vi "Get Feature Names.vi"(8 "error in (no error)":errorcluster caption="entrée d'erreur (pas d'erreur)", 9 "y":string[][](array[string]), 10 "X":string[][](array[string]), 11 "OneHotEncoder.lvclass":refnum<class "OneHotEncoder.lvclass">) -> (0 "error out":errorcluster caption="sortie d'erreur", 2 "Data":T1, 3 "OneHotEncoder.lvclass":refnum<class "OneHotEncoder.lvclass">)   [LabVIEW 2020, in "OneHotEncoder.lvclass"]
doc: "Return feature names for output features.\n\nReturns : \n\n- output_feature_names : ndarray of shape (n_output_features,)\nArray of feature names."
uses:
  OneHotEncoder.lvclass
  OneHotEncoder.lvclass/OneHotEncoder.ctl
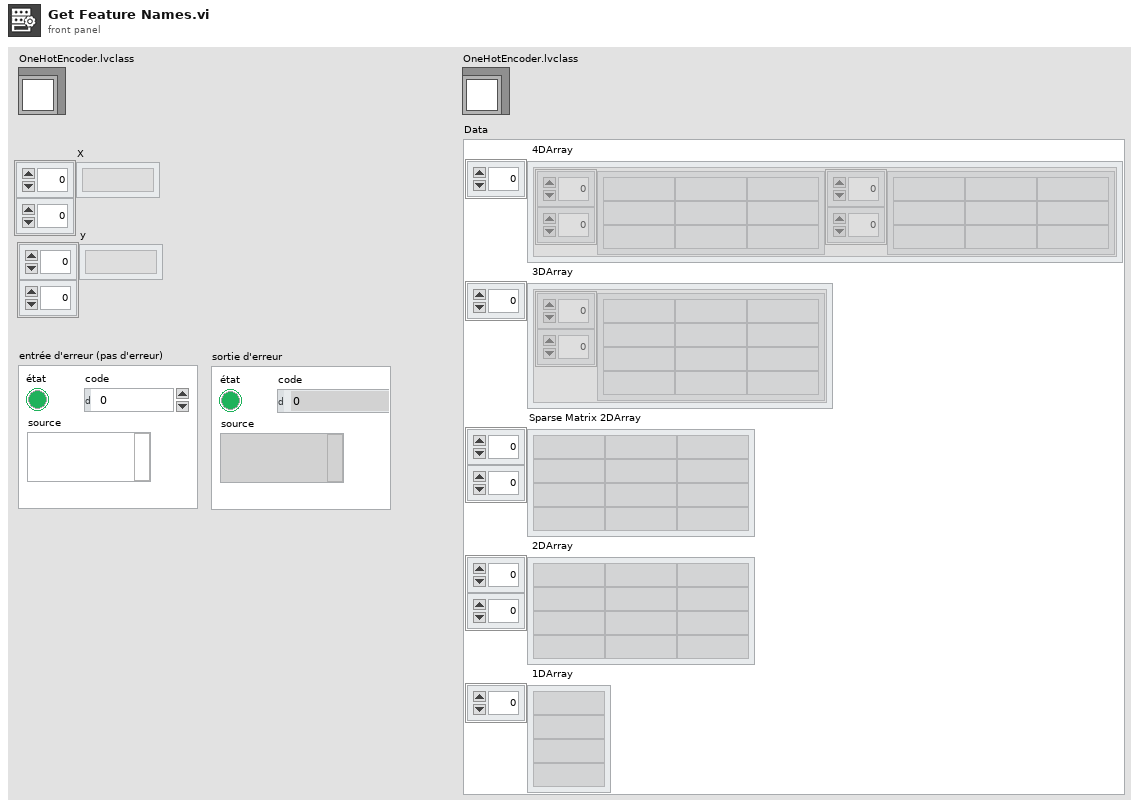
[diagram p1: front panel]
types:
  T1 = cluster{" 4DArray":cluster{"1":string[][], "2":string[][]}[], " 3DArray":cluster{"Tableau":string[][]}[], "Sparse Matrix 2DArray":string[][], " 2DArray":string[][], " 1DArray":string[]}
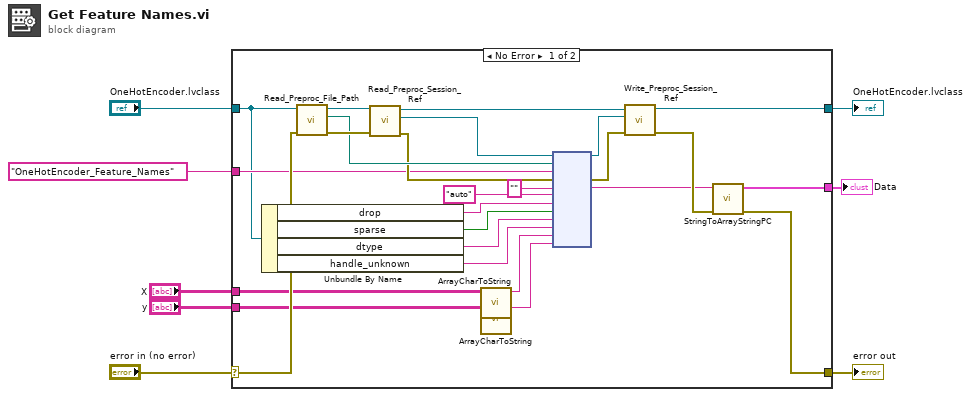
[diagram p0: block diagram]
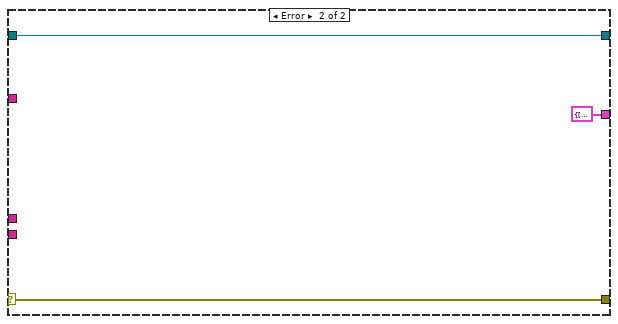
[diagram p2: hidden frame]
diagram:
  n1 = case shown="No Error" "error in (no error)" {
    selector: "error in (no error)" -> [w24 w37]
    tunnel: [w10 w37] -> w7
    tunnel: [w13 w36] -> w5
    tunnel: "OneHotEncoder.lvclass" -> [w22 w36]
    tunnel: "OneHotEncoder_Feature_Names" ("Fonction") -> [w23 _]
    tunnel: [w9 T1 {" 4DArray"=[], " 3DArray"=[], "Sparse Matrix 2DArray"=[], " 2DArray"=[], " 1DArray"=[]} ("Data")] -> w3
    tunnel: "X" -> [w17 _]
    tunnel: "y" -> [w16 _]
    frame No Error {
      n2 = Unbundle By Name(w22) -> ("drop"=w25:string, "sparse"=w20:bool, "dtype"=w19:string, "handle_unknown"=w18:string)
      n3 = call-dynamic "Read_Preproc_File_Path.vi"("error in (no error)"=w24, "Python in"=w22) -> ("error out"=w33:errorcluster, "File_Path"=w30:path, "Python out"=w34:refnum<class "OneHotEncoder.lvclass">)  [unwired: 7 in]
      n4 = call-dynamic "Read_Preproc_Session_Ref.vi"("error in (no error)"=w33, "Python in"=w34) -> ("error out"=w29:errorcluster, "Session_ref"=w31:refnum<k35>, "Python out"=w32:refnum<class "OneHotEncoder.lvclass">)  [unwired: 7 in]
      n5 = call "ArrayCharToString.vi"("TAB"=w17) -> ("Instruction"=w15:string)  [unwired: 10 in]
      n6 = call "ArrayCharToString.vi"("TAB"=w16) -> ("Instruction"=w14:string)  [unwired: 10 in]
      n7 = node(w31, w30, w23, w29, "", "auto", w25, w20, w19, w18, w15, w14) -> (w27:refnum<k35>, w28:errorcluster, w11:string)  [unwired: 7 in, 2 out]
      n8 = call-dynamic "Write_Preproc_Session_Ref.vi"("error in (no error)"=w28, "Session_ref"=w27, "Python in"=w32) -> ("error out"=w12:errorcluster, "Python out"=w13:refnum<class "OneHotEncoder.lvclass">)  [unwired: 7 in]
      n9 = call "StringToArrayStringPC.vi"("sortie d'erreur"=w12, "Return value"=w11) -> ("sortie d'erreur"=w10:errorcluster, "Data"=w9:T1)  [unwired: 8 in]
    }
    frame Error {
    }
  }
  "error out" <- w7
  "OneHotEncoder.lvclass" <- w5
  "Data" <- w3
